vi "perpendicularDist.vi"(5 "Y2":dbl, 7 "X1":dbl, 9 "C":dbl, 10 "B":dbl, 11 "A":dbl) -> (1 "Distance":dbl)   [LabVIEW 2016]
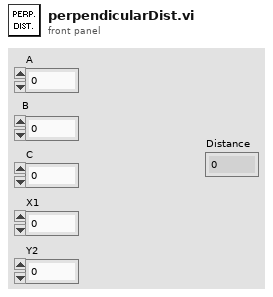
[diagram p1: front panel]
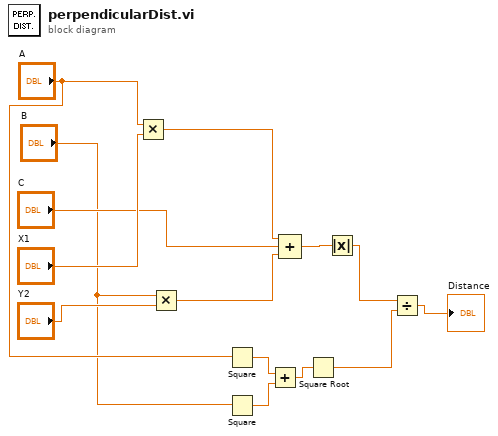
[diagram p0: block diagram]
diagram:
  n1 = Multiply(x="A", y="X1") -> (x*y=w12:dbl)
  n2 = Multiply(x="B", y="Y2") -> (x*y=w10:dbl)
  n3 = Square(x="A") -> (x^2=w6:dbl)
  n4 = Square(x="B") -> (x^2=w5:dbl)
  n5 = Add(x=w6, y=w5) -> (x+y=w4:dbl)
  n6 = Compound Arithmetic op=ADD(w12, "C", w10) -> (w9:dbl)
  n7 = Square Root(x=w4) -> (sqrt(x)=w2:dbl)
  n8 = Absolute Value(x=w9) -> (abs(x)=w3:dbl)
  n9 = Divide(x=w3, y=w2) -> (x/y=→"Distance":dbl)
